vi "I32.vi"(8 "Error In":errorcluster) -> (0 "Error Out":errorcluster)   [LabVIEW 2017, in "Tests.lvlib" / "From Msgpack.lvlib"]
uses:
  From Msgpack.lvlib
  <vilib>/addons/_JKI Toolkits/Caraya/classes/Test/Test.lvclass
  src/LabPack/LabPack.lvlib
  <vilib>/addons/_JKI Toolkits/Caraya/classes/Assert/Assert.lvclass
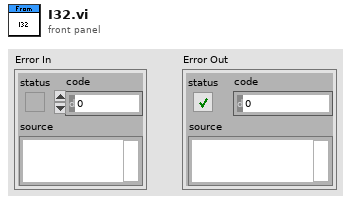
[diagram p1: front panel]
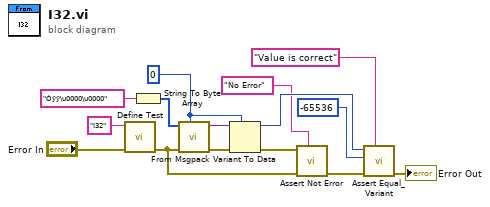
[diagram p0: block diagram]
diagram:
  w2 = 0
  n1 = call <vilib>:"Define Test.vi"("error in (no error)"="Error In", "Label (VI Title)"="I32") -> ("error out"=w8:errorcluster)  [unwired: 9 in]
  n2 = String To Byte Array(string="Òÿÿ\u0000\u0000") -> (unsigned byte array=w11:u8[])
  n3 = call "From Msgpack.vi"("Types and Defaults"=w2, "Error In"=w8, "Msgpack Data"=w11) -> ("Error Out"=w13:errorcluster, "Value"=w10:variant)  [unwired: 7 in]
  n4 = Variant To Data(error in=w13, type=w2, Variant=w10) -> (data=w5:i32, error out=w9:errorcluster)
  n5 = call <vilib>:"Assert Not Error.vi"("Label"="No Error", "error in (no error)"=w8, "Not Error?"=w9) -> ("error out"=w7:errorcluster)  [unwired: 8 in]
  n6 = call <vilib>:"Assert Equal_Variant.vi"("Label"="Value is correct", "error in (no error)"=w7, "Y"=-65536, "X"=w5) -> ("error out"=→"Error Out":errorcluster)  [unwired: 7 in]
